vi "Initiate External Data Log.vi"(8 "error in (no error)":errorcluster {"code" format="%.0x"}, 10 "Channel Name (1)":string="1", 11 "VISA resource name":refnum<visa-resource-name>) -> (0 "error out":errorcluster {"code" format="%.0x"}, 3 "VISA resource name out":refnum<visa-resource-name>)   [LabVIEW 2010, in "Agilent N6700 Series.lvlib"]
doc: "Initiates an external data log. When the external data log is initiated, an event on a selected external data log trigger source starts the data log. If the external data log is not initiated, all triggers are ignored.\n\n<b>Note:</b>\n\n(1) The external data log function is not accessible from the instrument's front panel.\n\n(2) All external data log functions are controlled using SCPI commands."
uses:
  Agilent N6700 Series.lvlib
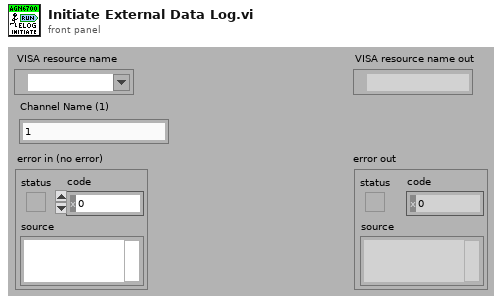
[diagram p1: front panel]
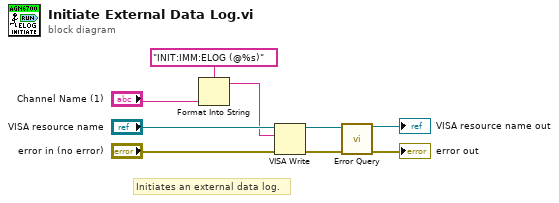
[diagram p0: block diagram]
diagram:
  # "Initiates an external data log."
  n1 = Format Into String(format string="INIT:IMM:ELOG (@%s)", "Channel Name (1)") -> (resulting string=w7:string)  [unwired: 2 in, 1 out]
  n2 = VISA Write(VISA resource name="VISA resource name", write buffer=w7, error in (no error)="error in (no error)") -> (VISA resource name out=w2:refnum<visa-resource-name>, error out=w1:errorcluster)  [unwired: 1 out]
  n3 = call "Error Query.vi"("VISA resource name"=w2, "error in (no error)"=w1) -> ("VISA resource name out"=→"VISA resource name out":refnum<visa-resource-name>, "error out"=→"error out":errorcluster)  [unwired: 10 in, 2 out]
